vi "Get Font.vi"(7 "Sheet Name":string, 8 "error in":errorcluster, 10 "Cell Address":string="A1", 11 "SpreadsheetDoc in":refnum<k24>) -> (0 "error out":errorcluster, 2 "Font":T1={"Bold"=enum."bold", "Italic"=enum."default", "Underline"=enum."none", "TextColor"=0, "TextSize"=-1.0, "Name"=""}, 3 "SpreadsheetDoc out":refnum<k24>)   [LabVIEW 2019, in "Open Xml.lvlib"]
uses:
  Open Xml.lvlib
  D:/git/Open-Xml-LabVIEW/Source/DocumentFormat.OpenXml.dll
  DocumentFormat.OpenXml.dll
  D:/git/Open-Xml-LabVIEW/Source/DocumentFormat.OpenXml.Framework.dll
  DocumentFormat.OpenXml.Framework.dll
  Font.ctl
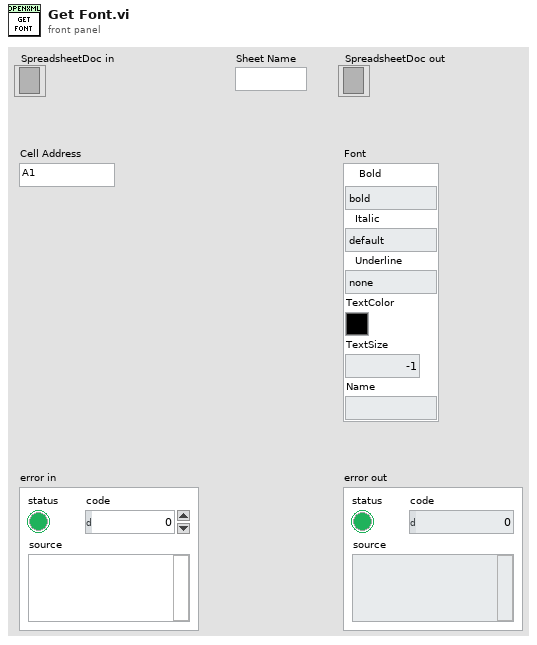
[diagram p1: front panel]
types:
  T1 = typedef "Open Xml.lvlib/Font.ctl" = cluster{"Bold":enum16{"bold", "regular", "default"}, "Italic":enum16{"italic", "regular", "default"}, "Underline":enum16{"single", "double", "singleAccounting", "doubleAccounting", "none", "default"}, "TextColor":u32, "TextSize":dbl, "Name":string}
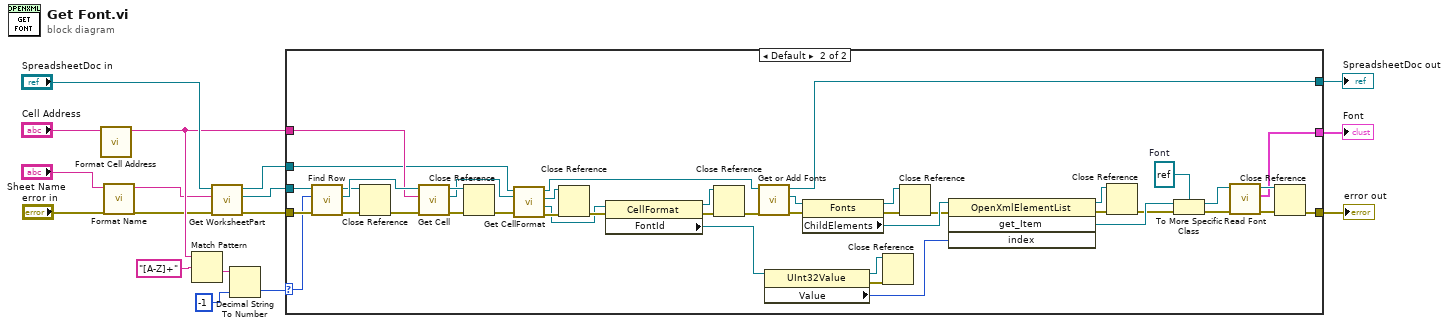
[diagram p0: block diagram]
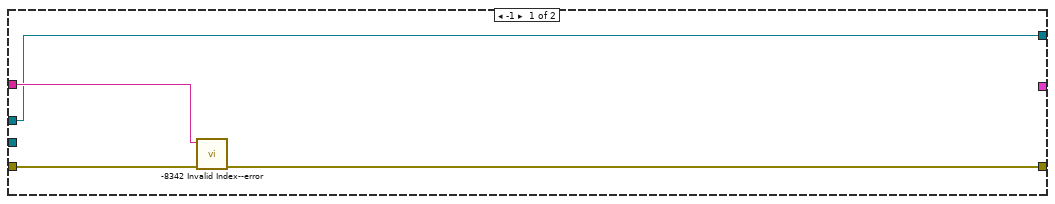
[diagram p2: hidden frame]
diagram:
  n1 = call "Format Cell Address.vi"("Cell Address"="Cell Address") -> ("Formatted Cell Address"=w4:string)  [unwired: 10 in]
  n2 = call "Format Name.vi"("Sheet Name"="Sheet Name") -> ("Formatted Sheet Name"=w1:string)  [unwired: 10 in]
  n3 = Match Pattern(string=w4, regular expression="[A-Z]+") -> (after substring=w9:string)  [unwired: 1 in, 3 out]
  n4 = call "Get WorksheetPart.vi"("error in"="error in", "Sheet Name"=w1, "SpreadsheetDoc in"="SpreadsheetDoc in") -> ("error out"=w14:errorcluster, "WorksheetPart"=w11:refnum<k24>, "SpreadsheetDoc out"=w12:refnum<k24>)  [unwired: 5 in, 1 out]
  n5 = Decimal String To Number(string=w9, default (0L)=i64 -1 ("default (0 I32)")) -> (number=w7:i64)  [unwired: 1 in, 1 out]
  n6 = case shown="Default" w7 {
    selector: w7 -> [_ w57]
    tunnel: [w17 w40] -> w16
    tunnel: [w19 w63] -> w15
    tunnel: w14 -> [w20 w60]
    tunnel: w12 -> [w17 w52]
    tunnel: w11 -> [_ w59]
    tunnel: w4 -> [w18 w56]
    tunnel: [_ w32] -> w6
    frame -1 {
      n7 = call "-8342 Invalid Index--error.vi"("error in"=w20, "Index"=w18) -> ("error out"=w19:errorcluster)  [unwired: 9 in]
    }
    frame Default {
      w35 = refnum<k24> refnum  # Font
      n8 = call "Find Row.vi"("error in"=w60, "Row Index"=w57, "Worksheetpart in"=w59) -> ("error out"=w61:errorcluster, "Row"=w58:refnum<k24>, "WorksheetPart out"=w54:refnum<k24>)  [unwired: 6 in]
      n9 = Close Reference(reference=w54, error in (no error)=w61) -> (error out=w55:errorcluster)
      n10 = call "Get Cell.vi"("error in"=w55, "Cell Address"=w56, "Row in"=w58) -> ("error out"=w62:errorcluster, "Cell"=w25:refnum<k24>, "Row out"=w53:refnum<k24>)  [unwired: 6 in]
      n11 = Close Reference(reference=w53, error in (no error)=w62) -> (error out=w26:errorcluster)
      n12 = call "Get CellFormat.vi"("error in"=w26, "Cell In"=w25, "SpreadsheetDoc in"=w52) -> ("error out"=w51:errorcluster, "CellFormat"=w48:refnum<k24>, "Cell out"=w50:refnum<k24>, "SpreadsheetDoc out"=w41:refnum<k24>)  [unwired: 5 in]
      n13 = Close Reference(reference=w50, error in (no error)=w51) -> (error out=w49:errorcluster)
      n14 = property class="CellFormat"(reference=w48, error in=w49) -> (reference out=w23:refnum<k24>, error out=w43:errorcluster, "FontId"=w30:refnum<k24>)
      n15 = Close Reference(reference=w23, error in (no error)=w43) -> (error out=w24:errorcluster)
      n16 = call "Get or Add Fonts.vi"("error in"=w24, "SpreadsheetDoc in"=w41) -> ("error out"=w46:errorcluster, "Fonts"=w47:refnum<k24>, "SpreadsheetDoc out"=w40:refnum<k24>)  [unwired: 7 in]
      n17 = property class="UInt32Value"(reference=w30) -> (reference out=w27:refnum<k24>, error out=w28:errorcluster, "Value"=w29:u32)  [unwired: 1 in]
      n18 = property class="Fonts"(reference=w47, error in=w46) -> (reference out=w36:refnum<k24>, error out=w44:errorcluster, "ChildElements"=w45:refnum<k24>)
      n19 = Close Reference(reference=w27, error in (no error)=w28) -> ()  [unwired: 1 out]
      n20 = Close Reference(reference=w36, error in (no error)=w44) -> (error out=w37:errorcluster)
      n21 = invoke class="OpenXmlElementList" method="get_Item"(reference=w45, error in=w37, "index"=w29) -> (reference out=w21:refnum<k24>, error out=w42:errorcluster, "get_Item"=w38:refnum<k24>)  [unwired: 1 in, 1 out]
      n22 = Close Reference(reference=w21, error in (no error)=w42) -> (error out=w22:errorcluster)
      n23 = To More Specific Class(target class=w35, reference=w38, error in=w22) -> (specific class reference=w34:refnum<k24>, error out=w39:errorcluster)
      n24 = call "Read Font.vi"("error in"=w39, "Font in"=w34) -> ("error out"=w31:errorcluster, "Font"=w32:T1, "Font out"=w33:refnum<k24>)  [unwired: 7 in]
      n25 = Close Reference(reference=w33, error in (no error)=w31) -> (error out=w63:errorcluster)
    }
  }
  "SpreadsheetDoc out" <- w16
  "error out" <- w15
  "Font" <- w6
